vi "Configure Trigger.vi"(0 "VISA resource name":refnum<visa-resource-name>, 1 "Enable Auto Trigger Delay (T: Enable)":bool=TRUE, 2 "Manual Trigger Delay (4 ms)":dbl=0.004, 5 "Trigger Source (0: Immediate)":u16(ring) items=["Immediate", "Video", "Line", "RF Burst", "TV", "External1", "External2"], 7 "Trigger Slope (0: Positive)":u16(ring) items=["Positive", "Negative"], 11 "error in (no error)":errorcluster, 12 "Enable Auto Trigger Offset (Disable)":bool, 13 "Manual Trigger Offset (4 ms)":dbl=0.004) -> (4 "VISA resource name out":refnum<visa-resource-name>, 15 "error out":errorcluster)   [LabVIEW 2014, in "Agilent ESA PSA Series.lvlib"]
doc: "Configures the trigger settings on the spectrum analyzer."
uses:
  Agilent ESA PSA Series.lvlib
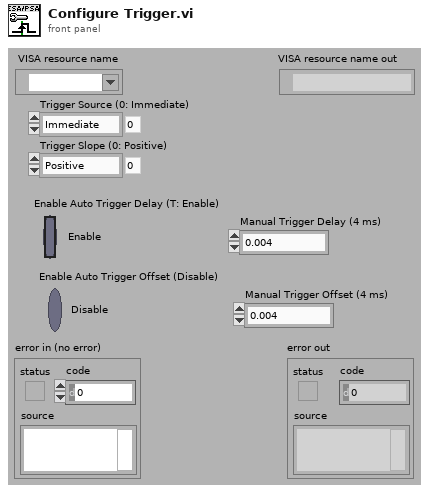
[diagram p1: front panel]
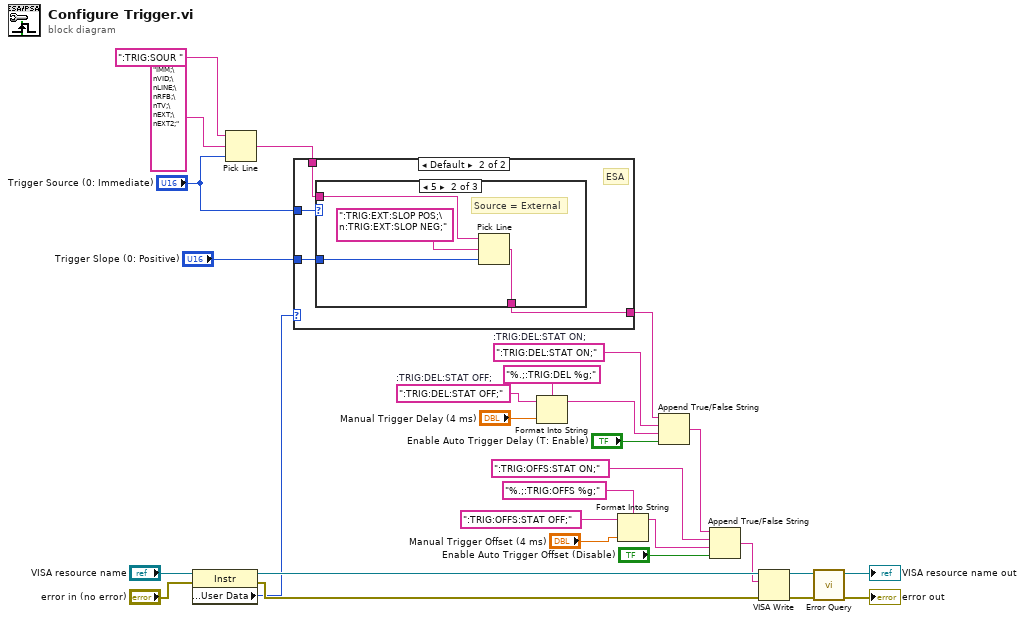
[diagram p0: block diagram]
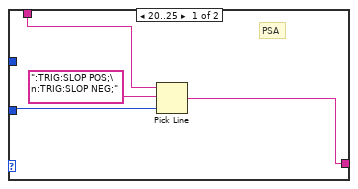
[diagram p2: hidden frame]
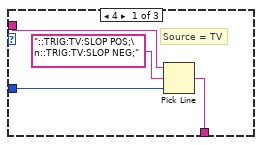
[diagram p3: hidden frame]
diagram:
  w10 = ":TRIG:DEL:STAT ON;"  # :TRIG:DEL:STAT ON;
  w12 = ":TRIG:DEL:STAT OFF;"  # :TRIG:DEL:STAT OFF;
  n1 = property class="Instr"(reference="VISA resource name", error in="error in (no error)") -> (reference out=w20:refnum<visa-resource-name>, error out=w21:errorcluster, "General Settings:User Data"=w19:u32)
  n2 = Pick Line(string ("")=":TRIG:SOUR ", multi-line string="IMM;\nVID;\nLINE;\nRFB;\nTV;\nEXT;\nEXT2;", line index="Trigger Source (0: Immediate)") -> (output string=w16:string)
  n3 = case shown="Default" w19 {
    tunnel: "Trigger Source (0: Immediate)" -> [_ w37]
    tunnel: "Trigger Slope (0: Positive)" -> [w32 w36]
    tunnel: w16 -> [w31 w35]
    tunnel: [w30 w34] -> w5
    frame 20..25 {
      # "PSA"
      n4 = Pick Line(string ("")=w31, multi-line string=":TRIG:SLOP POS;\n:TRIG:SLOP NEG;", line index=w32) -> (output string=w30:string)
    }
    frame Default {
      # "ESA"
      n5 = case shown="5" w37 {
        tunnel: [w40 w44 w46] -> w34
        tunnel: w36 -> [w39 w43 _]
        tunnel: w35 -> [w38 w42 w46]
        frame 4 {
          # "Source = TV"
          n6 = Pick Line(string ("")=w38, multi-line string="::TRIG:TV:SLOP POS;\n::TRIG:TV:SLOP NEG;", line index=w39) -> (output string=w40:string)
        }
        frame 5 {
          # "Source = External"
          n7 = Pick Line(string ("")=w42, multi-line string=":TRIG:EXT:SLOP POS;\n:TRIG:EXT:SLOP NEG;", line index=w43) -> (output string=w44:string)
        }
        frame Default {
        }
      }
    }
  }
  n8 = Format Into String(format string="%.;:TRIG:DEL %g;", initial string=w12, "Manual Trigger Delay (4 ms)") -> (resulting string=w11:string)  [unwired: 1 in, 1 out]
  n9 = Format Into String(format string="%.;:TRIG:OFFS %g;", initial string=":TRIG:OFFS:STAT OFF;", "Manual Trigger Offset (4 ms)") -> (resulting string=w2:string)  [unwired: 1 in, 1 out]
  n10 = Append True/False String(1:"Enable Auto Trigger Delay (T: Enable)", 2:w11, 3:w10, 4:w5) -> (0:w4:string)
  n11 = Append True/False String(1:"Enable Auto Trigger Offset (Disable)", 2:w2, 3:":TRIG:OFFS:STAT ON;" ("initial string"), 4:w4) -> (0:w3:string)
  n12 = VISA Write(VISA resource name=w20, write buffer=w3, error in (no error)=w21) -> (VISA resource name out=w29:refnum<visa-resource-name>, error out=w27:errorcluster)  [unwired: 1 out]
  n13 = call "Error Query.vi"("error in (no error)"=w27, "VISA resource name"=w29) -> ("error out"=→"error out":errorcluster, "VISA resource name out"=→"VISA resource name out":refnum<visa-resource-name>)  [unwired: 6 in, 2 out]
